vi "Format Columns.vi"(8 "error in (no error)":errorcluster, 11 "ORM Scripter in":refnum<class "ORM Scripter.lvclass">) -> (0 "error out":errorcluster, 2 "String":string, 3 "ORM Scripter out":refnum<class "ORM Scripter.lvclass">)   [LabVIEW 2018, in "ORM Scripter.lvclass"]
uses:
  ORM Scripter.lvclass
  ORM Scripter.lvclass/ORM Scripter.ctl
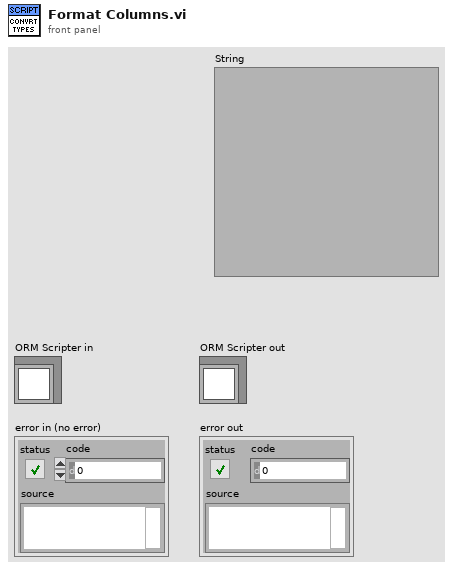
[diagram p1: front panel]
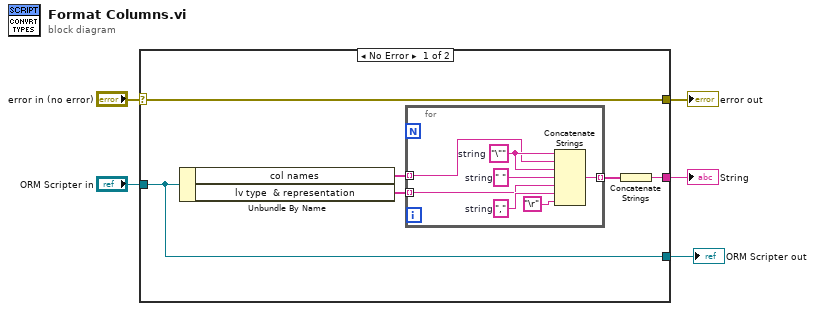
[diagram p0: block diagram]
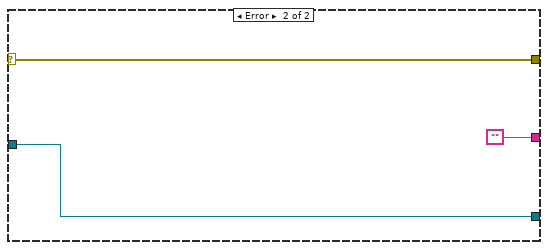
[diagram p2: hidden frame]
diagram:
  n1 = case shown="No Error" "error in (no error)" {
    selector: "error in (no error)" -> [w9 w21]
    tunnel: "ORM Scripter in" -> [w6 w20]
    tunnel: [w9 w21] -> w3
    tunnel: [w7 ""] -> w2
    tunnel: [w6 w20] -> w1
    frame No Error {
      n2 = Unbundle By Name(w6) -> ("col names"=w11:string[], "lv type  & representation"=w10:string[])
      n3 = for {
        tunnel: [w17] -> w8 mode=indexing
        tunnel: w11 -> [w13] mode=indexing
        tunnel: w10 -> [w12] mode=indexing
        w16 = ","  # string
        w15 = " "  # string
        w14 = "\""  # string
        n4 = Concatenate Strings(w14, w13, w14, w15, w12, w16, "\r") -> (w17:string)
      }
      n5 = Concatenate Strings(w8) -> (w7:string)
    }
    frame Error {
    }
  }
  "String" <- w2
  "error out" <- w3
  "ORM Scripter out" <- w1
